vi "Init.vi"(0 "InterfaceLog in":refnum<class "InterfaceLog.lvclass">, 1 "Log Path":path, 3 "error in (no error)":errorcluster) -> (7 "InterfaceLog out":refnum<class "InterfaceLog.lvclass">, 10 "error out":errorcluster)   [LabVIEW 2016, in "InterfaceLog.lvclass"]
uses:
  InterfaceLog.lvclass
  InterfaceLog.lvclass/InterfaceLog.ctl
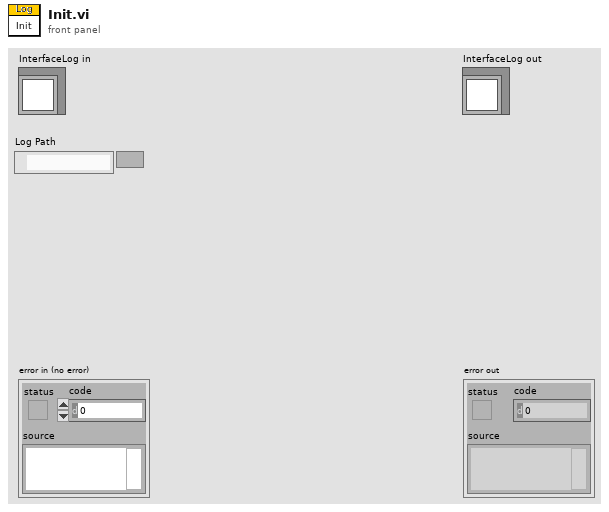
[diagram p1: front panel]
types:
  T1 = enum16{"open", "replace", "create", "open or create", "replace or create", "replace or create with confirmation"}
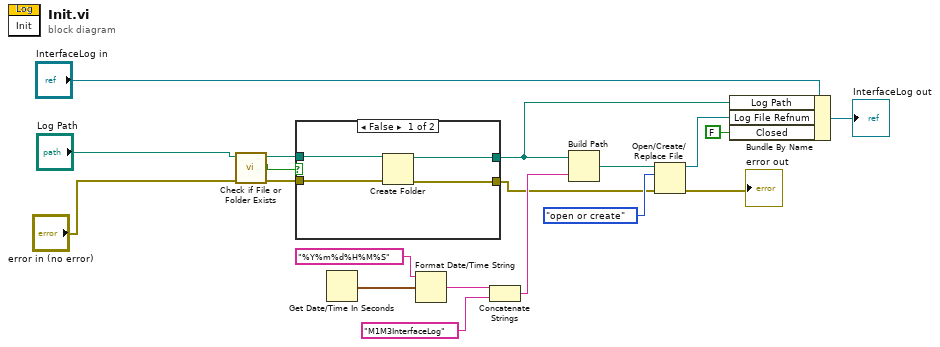
[diagram p0: block diagram]
diagram:
  n1 = call <vilib>:"Check if File or Folder Exists.vi"("error in (no error)"="error in (no error)", "path"="Log Path") -> ("error out"=w17:errorcluster, "file or folder exists?"=w19:bool, "dup path"=w16:path)  [unwired: 7 in]
  n2 = case shown="False" w19 {
    tunnel: w17 -> [w22 w24]
    tunnel: w16 -> [w23 w25]
    tunnel: [w21 w25] -> w5
    tunnel: [w20 w24] -> w8
    frame False {
      n3 = Create Folder(path (use dialog)=w23, error in=w22) -> (created path=w21:path, error out=w20:errorcluster)  [unwired: 1 in, 1 out]
    }
    frame True {
    }
  }
  n4 = Get Date/Time In Seconds() -> (seconds since 1Jan1904=w15:timestamp)
  n5 = Format Date/Time String(time format string (%c)="%Y%m%d%H%M%S", seconds (now)=w15) -> (date/time string=w13:string)  [unwired: 1 in]
  n6 = Concatenate Strings(w13, "M1M3InterfaceLog" ("string")) -> (w11:string)
  n7 = Build Path(base path=w5, name or relative path=w11) -> (appended path=w10:path)
  n8 = Open/Create/Replace File(file path (use dialog)=w10, error in=w8, operation (0:open)=T1."open or create") -> (refnum out=w4:refnum<file>, error out=→"error out":errorcluster)  [unwired: 3 in, 1 out]
  n9 = Bundle By Name(cluster="InterfaceLog in", "Log Path"=w5, "Log File Refnum"=w4, "Closed"=FALSE) -> (→"InterfaceLog out":refnum<class "InterfaceLog.lvclass">)
